vi "Set Grating.vi"(8 "error in (no error)":errorcluster, 10 "NEW GRT?":u8=1 min=1 max=3 step=1, 11 "VISA resource name":refnum<visa-resource-name>) -> (0 "error out":errorcluster, 3 "VISA resource name out":refnum<visa-resource-name>)   [LabVIEW 2012, in "Digikrom DK24x.lvlib"]
doc: "This command changes gratings, if additional gratings are installed."
uses:
  Digikrom DK24x.lvlib
  Private/Command.ctl
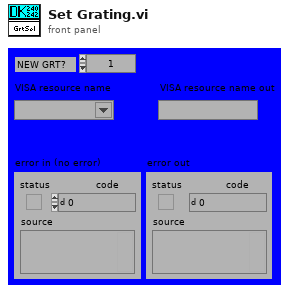
[diagram p1: front panel]
types:
  T1 = typedef "Digikrom DK24x.lvlib/Command.ctl" = u8
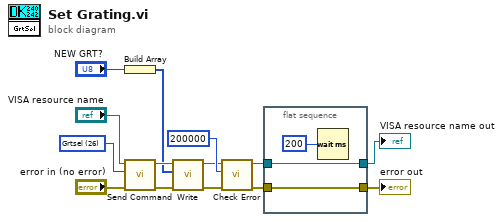
[diagram p0: block diagram]
diagram:
  w5 = T1 26 items=["Cancel"=24, "Clear"=25, "CSR"=28, "Echo"=27, "Filter"=15, "Gcal"=18, "Goto"=16, "Grtid?"=19, "Grtsel"=26, "NOVRAM Read"=56, "NOVRAM Write"=59, "Reset"=255, "Scan"=12, "Scan Up"=9, "Scan Down"=3, "Serial?"=33, "Slew Up"=8, "Slew Down"=2, "Slit Reset"=43, "Slit?"=30, "Sltadj"=14, "Speed"=13, "Sspeed?"=21, "Step Down"=1, "Step Up"=7, "S1adj"=31, "S2adj"=32, "S3adj"=34, "S1cal"=22, "S2cal"=23, "S3cal"=35, "Test"=17, "Type"=57, "Wave?"=29, "Zero"=52] ("Command")
  n1 = Build Array("NEW GRT?") -> (w6:u8[])
  n2 = call "Send Command.vi"("error in (no error)"="error in (no error)", "Command"=w5, "VISA resource name"="VISA resource name") -> ("error out"=w9:errorcluster, "VISA resource name out"=w10:refnum<visa-resource-name>)  [unwired: 7 out]
  n3 = call "Write.vi"("error in (no error)"=w9, "Byte Array"=w6, "VISA resource name"=w10) -> ("error out"=w12:errorcluster, "VISA resource name out"=w11:refnum<visa-resource-name>)  [unwired: 7 out]
  n4 = call "Check Error.vi"("error in"=w12, "timeout"=u32 200000, "VISA resource name in"=w11) -> ("error out"=w2:errorcluster, "VISA resource name out"=w4:refnum<visa-resource-name>)  [unwired: 7 out]
  n5 = flat-sequence {
    tunnel: w4 -> [w16]
    tunnel: [w16] -> w3
    tunnel: w2 -> [w15]
    tunnel: [w15] -> w1
    frame #0 {
      n6 = Wait (ms)(milliseconds to wait=u32 200) -> ()  [unwired: 1 out]
    }
  }
  "error out" <- w1
  "VISA resource name out" <- w3
